vi "PickedPoint.vi"(8 "error in (no error)":errorcluster, 10 "Point":T2, 11 "Render Window in":refnum<class "Render Window.lvclass">) -> (0 "error out":errorcluster, 1 "Hit?":bool, 2 "PickPoint":T1, 3 "Render Window out":refnum<class "Render Window.lvclass">)   [LabVIEW 2015, in "Render Window.lvclass"]
uses:
  Render Window.lvclass
  <vilib>/Utility/miscctls.llb/LVPoint32TypeDef.ctl
  <vilib>/Utility/miscctls.llb/LV3DPointTypeDef.ctl
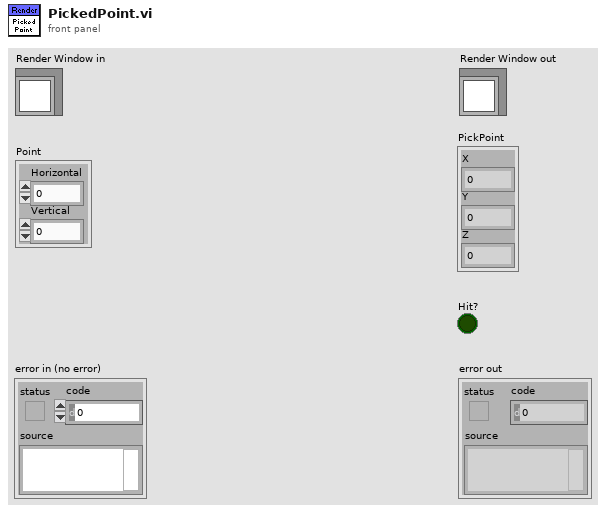
[diagram p1: front panel]
types:
  T1 = typedef "LV3DPointTypeDef.ctl" = cluster{"X":sgl, "Y":sgl, "Z":sgl}
  T2 = typedef "LVPoint32TypeDef.ctl" = cluster{"Horizontal":i32, "Vertical":i32}
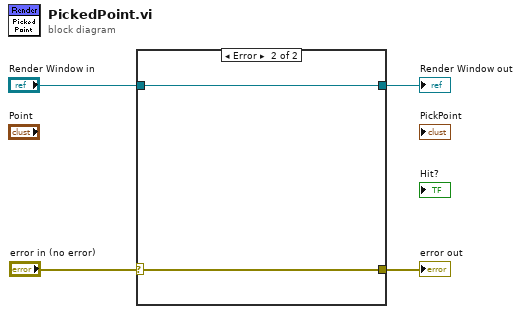
[diagram p0: block diagram]
diagram:
  n1 = case shown="Error" "error in (no error)" {
    selector: "error in (no error)" -> [w6 w8]
    tunnel: [w6 w8] -> w3
    tunnel: [w5 w7] -> w2
    tunnel: "Render Window in" -> [w5 w7]
    frame No Error {
    }
    frame Error {
    }
  }
  "error out" <- w3
  "Render Window out" <- w2
